vi "Trigger Display Mode.vi"(8 "Error In":errorcluster, 9 "Display Mode":string, 10 "Duration(ms)":u32, 11 "Sequencer In":refnum<class "Sequencer.lvclass">) -> (0 "Error Out":errorcluster, 3 "Sequencer Out":refnum<class "Sequencer.lvclass">)   [LabVIEW 2021, in "Sequencer.lvclass"]
uses:
  Sequencer.lvclass
  C:/Git/MEMOSFET/myDashBoard/Source/RT/Process/Process.lvclass
  Central Message Handler/Public/Controls/Message.ctl
  Central Message Handler/Central Message Handler.lvclass
  Process/Process.lvclass
  Utilities/Utilities.lvlib
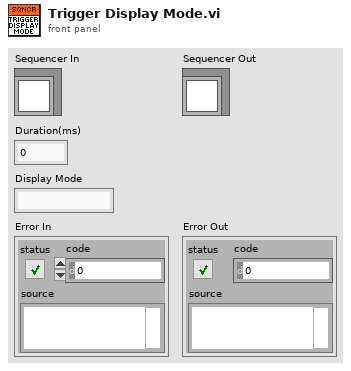
[diagram p1: front panel]
types:
  T1 = typedef "Central Message Handler.lvclass/Message.ctl" = cluster{"Command":string, "Data":variant, "Receiver":string}
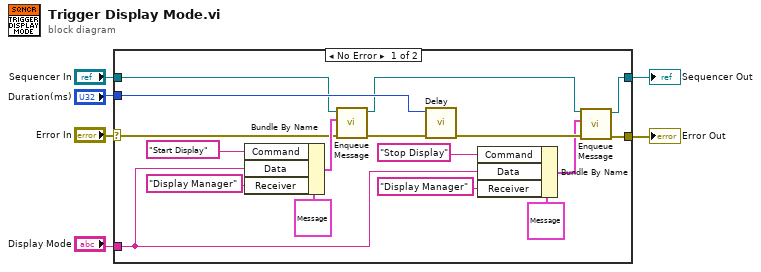
[diagram p0: block diagram]
diagram:
  n1 = case shown="No Error" "Error In" {
    selector: "Error In" -> [w9 w24]
    tunnel: "Duration(ms)" -> [w22 _]
    tunnel: [w20 w24] -> w5
    tunnel: [w15 w25] -> w4
    tunnel: "Display Mode" -> [w7 _]
    tunnel: "Sequencer In" -> [w8 w25]
    frame No Error {
      n2 = Bundle By Name(cluster=T1 {"Command"="Start Display", "Data"=variant, "Receiver"="Display Manager"} ("Message"), "Command"="Start Display", "Data"=w7, "Receiver"="Display Manager") -> (w13:T1)
      n3 = call "Enqueue Message.vi"("Error In"=w9, "Message"=w13, "Process In"=w8) -> ("Error Out"=w21:errorcluster, "Process Out"=w14:refnum<class "Sequencer.lvclass">)  [unwired: 7 in]
      n4 = call "Delay.vi"("Error In"=w21, "Milliseconds To Wait"=w22) -> ("Error Out"=w23:errorcluster)  [unwired: 9 in]
      n5 = Bundle By Name(cluster=T1 {"Command"="Start Display", "Data"=variant, "Receiver"="Display Manager"} ("Message"), "Command"="Stop Display", "Data"=w7, "Receiver"="Display Manager") -> (w17:T1)
      n6 = call "Enqueue Message.vi"("Error In"=w23, "Message"=w17, "Process In"=w14) -> ("Error Out"=w20:errorcluster, "Process Out"=w15:refnum<class "Sequencer.lvclass">)  [unwired: 7 in]
    }
    frame Error {
    }
  }
  "Error Out" <- w5
  "Sequencer Out" <- w4
